vi "DSF.Engine.Interface.Transceiver.Read.Command.vi"(8 "error in (no error)":errorcluster, 9 "timeout in ms (0)":i32, 11 "Transceiver Interface in":refnum<class "DSF.Engine.Interface.Transceiver.lvclass">) -> (0 "error out":errorcluster, 1 "empty?":bool, 2 "command":T1, 3 "Transceiver Interface out":refnum<class "DSF.Engine.Interface.Transceiver.lvclass">, 4 "# elements":u32)   [LabVIEW 2017, in "DSF.Engine.lvlib" / "DSF.Engine.Interface.Transceiver.lvclass"]
uses:
  DSF.Engine.Interface.Transceiver.lvclass
  C:/Git/DSF/Source/Engine/Classes/Interface/DSF.Engine.Interface.lvclass
  DSF.Engine.Interface.Transceiver.Command Data.ctl
  DSF.Engine.Interface.Transceiver.Command.ctl
  DSF.Engine.Interface.Transceiver.Command Parameters.ctl
  DSF.Engine.Interface.lvclass/DSF.Engine.Interface.ctl
  DSF.Engine.Interface.lvclass
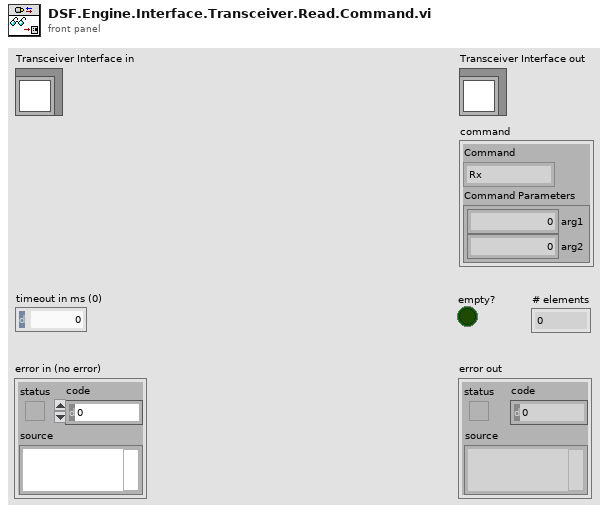
[diagram p1: front panel]
types:
  T1 = typedef "DSF.Engine.lvlib/DSF.Engine.Interface.Transceiver.lvclass/DSF.Engine.Interface.Transceiver.Command Data.ctl" = cluster{"Command":T2, "Command Parameters":T3}
  T2 = typedef "DSF.Engine.lvlib/DSF.Engine.Interface.Transceiver.lvclass/DSF.Engine.Interface.Transceiver.Command.ctl" = enum8{"Rx", "Tx", "Shutdown"}
  T3 = typedef "DSF.Engine.lvlib/DSF.Engine.Interface.Transceiver.lvclass/DSF.Engine.Interface.Transceiver.Command Parameters.ctl" = cluster{"arg1":u64, "arg2":u64}
  T4 = typedef "DSF.Engine.lvlib/DSF.Engine.Interface.lvclass/DSF.Engine.Interface.RT FIFO.Ref.16B.ctl" = refnum<k33>
  T5 = typedef "DSF.Engine.lvlib/DSF.Engine.Interface.lvclass/DSF.Engine.Interface.RT FIFO.Data.16B.ctl" = cluster{"Command":u8, "Payload":T6}
  T6 = typedef "DSF.Engine.lvlib/DSF.Engine.Interface.lvclass/DSF.Engine.Interface.RT FIFO.Payload.16B.ctl" = cluster{"arg1":u64, "arg2":u64}
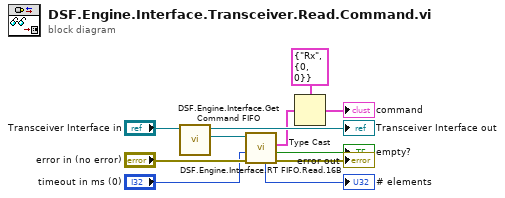
[diagram p0: block diagram]
diagram:
  n1 = call "DSF.Engine.Interface.Get Command FIFO.vi"("Interface in"="Transceiver Interface in") -> ("Command FIFO"=w10:T4, "Interface out"=→"Transceiver Interface out":refnum<class "DSF.Engine.Interface.Transceiver.lvclass">)  [unwired: 9 in]
  n2 = call "DSF.Engine.Interface.RT FIFO.Read.16B.vi"("error in (no error)"="error in (no error)", "timeout in ms (0)"="timeout in ms (0)", "RT FIFO in"=w10) -> ("error out"=→"error out":errorcluster, "empty?"=→"empty?":bool, "element out"=w5:T5, "# elements"=→"# elements":u32)  [unwired: 4 in, 1 out]
  n3 = Type Cast(type=T1 {"Command"=enum."Rx", "Command Parameters"={"arg1"=0, "arg2"=0}} ("Plugin Command"), x=w5) -> (*(type *) &x=→"command":T1)
